vi "sombrero.vi"() -> ()   [LabVIEW 2011]
uses:
  <vilib>/Math Plots/3D Math Plots/3D Surface/3D Surface XCtrl/3D Surface.xctl
  <vilib>/Math Plots/3D Math Plots/3D Surface/3D Surface Datatype/Public/Plot Helper (Vector).vi
  <vilib>/Math Plots/3D Math Plots/3D Surface/3D Surface Datatype/3D Surface Datatype.lvclass
panel:
  in  "Animaatio":bool
  in  "Voimakkuus":dbl(knob) scale=1.1..200.0
  in  "Aallonpituus":dbl(knob) scale=1.1..30.0
  out "3D Surface":refnum<class "3D Plot Datatype.lvclass">[](xcontrol)
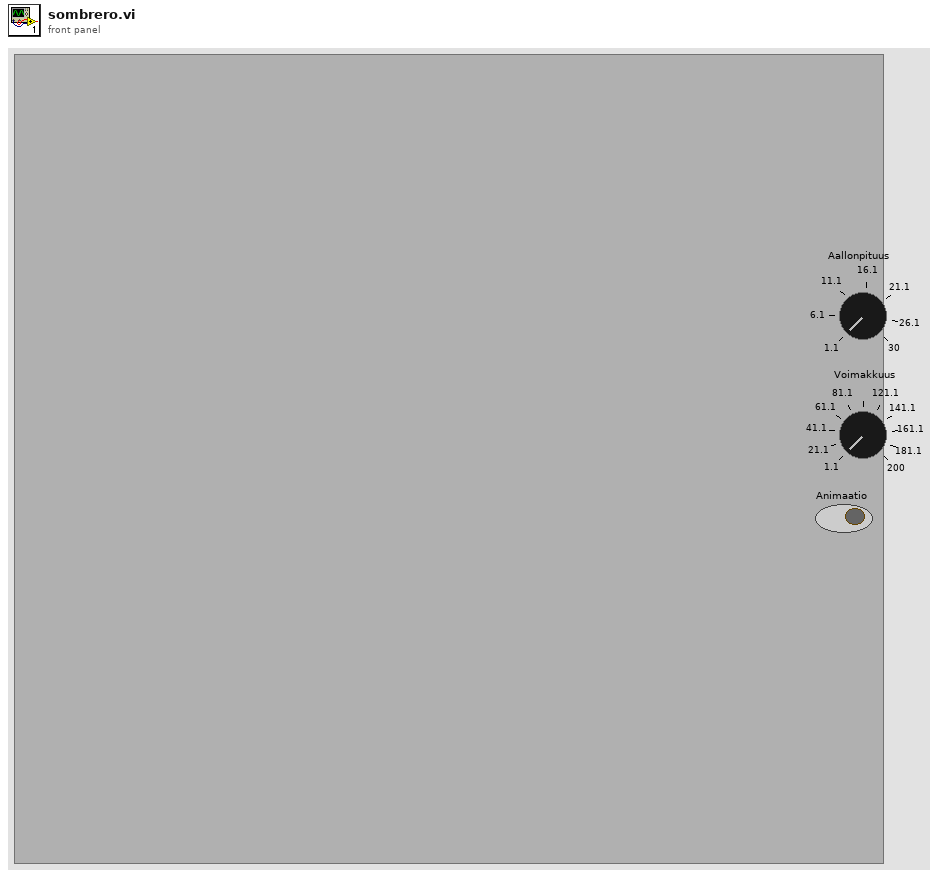
[diagram p1: front panel]
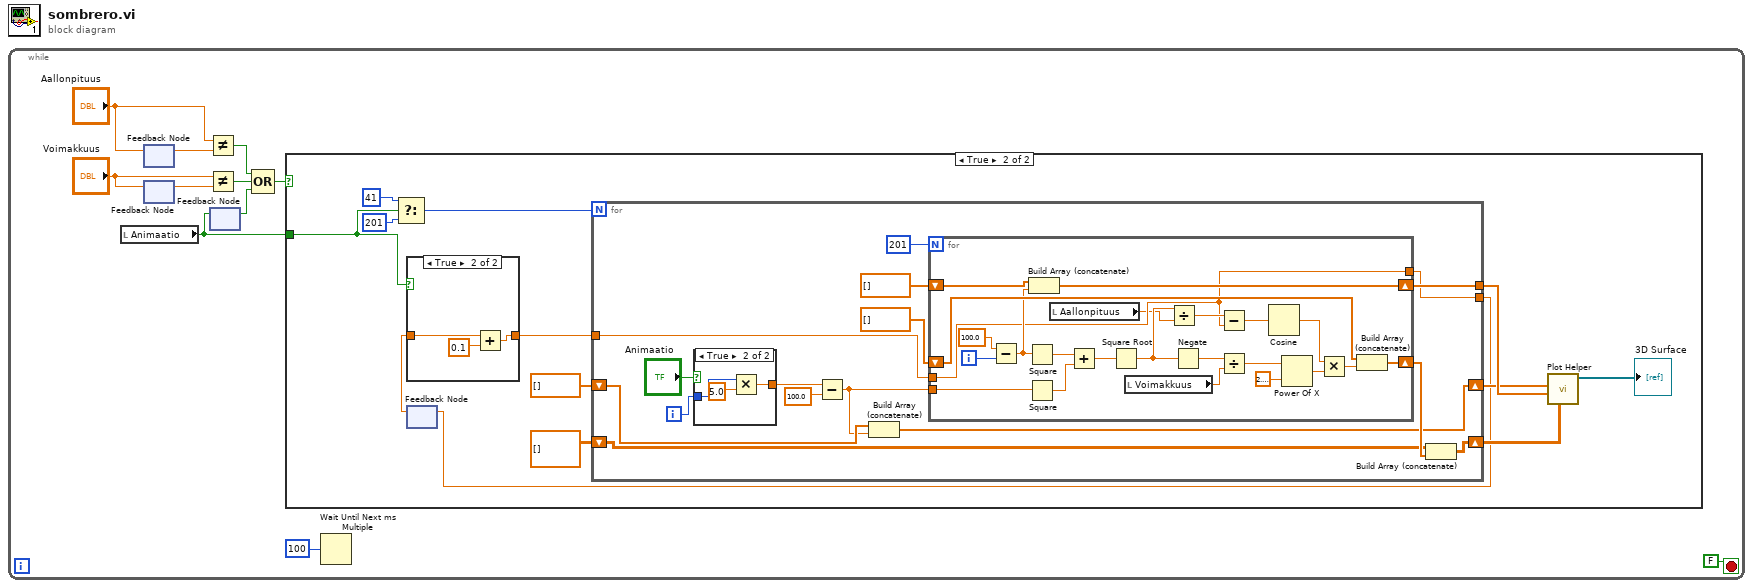
[diagram p0: block diagram]
diagram:
  n1 = while {
    stop <- FALSE stop-if-true
    n2 = local read "Animaatio"() -> (w5:bool)
    n3 = feedback-in #1("Aallonpituus") -> ()
    n4 = feedback #1() -> (w7:dbl)  [unwired: 1 in]
    n5 = feedback-in #2("Voimakkuus") -> ()
    n6 = feedback #2() -> (w9:dbl)  [unwired: 1 in]
    n7 = Not Equal?(x="Aallonpituus", y=w7) -> (x != y?=w4:bool)
    n8 = Not Equal?(x="Voimakkuus", y=w9) -> (x != y?=w3:bool)
    n9 = feedback-in #3(w5) -> ()
    n10 = feedback #3() -> (w2:bool)  [unwired: 1 in]
    n11 = Compound Arithmetic op=OR(w4, w3, w2) -> (w1:bool)
    n12 = case shown="True" w1 {
      tunnel: w5 -> [_ w16]
      frame False {
      }
      frame True {
        n13 = Select(t=41, s=w16, f=201) -> (s? t:f=w17:i32)
        n14 = feedback #4() -> (w12:dbl)  [unwired: 1 in]
        n15 = case shown="True" w16 {
          tunnel: [w25 w27] -> w20
          tunnel: w12 -> [w25 w26]
          frame False {
          }
          frame True {
            n16 = Add(x=w26, y=0.1) -> (x+y=w27:dbl)
          }
        }
        n17 = for {
          N: w17 -> [_]
          tunnel: [w38] -> w22
          shift-right: [w39] -> w23
          shift-left: dbl[][] [] -> [w42]
          tunnel: w20 -> [w37]
          tunnel: [w36] -> w13
          shift-right: [w34] -> w21
          shift-left: dbl[] [] -> [w35]
          i -> [w33]
          n18 = case shown="True" "Animaatio" {
            tunnel: w33 -> [w45 w47]
            tunnel: [w45 w46] -> w31
            frame False {
            }
            frame True {
              n19 = Multiply(x=w47, y=5.0) -> (x*y=w46:dbl)
            }
          }
          n20 = Subtract(x=w31, y=100.0) -> (x-y=w30:dbl)
          n21 = Build Array (concatenate)(w35, w30) -> (w34:dbl[])
          n22 = for {
            N: 201 -> [_]
            tunnel: w30 -> [w55]
            shift-right: [w66] -> w38
            shift-left: dbl[] [] -> [w65]
            shift-right: [w63] -> w43
            shift-left: dbl[] [] -> [w64]
            tunnel: w37 -> [w53]
            tunnel: [w53] -> w36
            i -> [w60]
            n23 = Subtract(x=100.0, y=w60) -> (x-y=w56:dbl)
            n24 = Square(x=w56) -> (x^2=w71:dbl)
            n25 = Square(x=w55) -> (x^2=w59:dbl)
            n26 = Build Array (concatenate)(w65, w56) -> (w66:dbl[])
            n27 = local read "Aallonpituus"() -> (w49:dbl)
            n28 = Add(x=w71, y=w59) -> (x+y=w70:dbl)
            n29 = Square Root(x=w70) -> (sqrt(x)=w68:dbl)
            n30 = local read "Voimakkuus"() -> (w51:dbl)
            n31 = Divide(x=w68, y=w49) -> (x/y=w54:dbl)
            n32 = Negate(x=w68) -> (-x=w69:dbl)
            n33 = Subtract(x=w54, y=w53) -> (x-y=w52:dbl)
            n34 = Divide(x=w69, y=w51) -> (x/y=w62:dbl)
            n35 = Cosine(x=w52) -> (cos(x)=w57:dbl)
            n36 = Power Of X(1:2.718281828459045, 2:w62) -> (0:w67:dbl)
            n37 = Multiply(x=w57, y=w67) -> (x*y=w58:dbl)
            n38 = Build Array (concatenate)(w64, w58) -> (w63:dbl[])
          }
          n39 = Build Array (concatenate)(w42, w43) -> (w39:dbl[][])
        }
        n40 = feedback-in #4(w13) -> ()
        n41 = call-poly <vilib>:"Plot Helper.vi"("z matrix"=w23, "y vector"=w22, "x vector"=w21) -> ("3D Plot lvclass Array out"=→"3D Surface":refnum<class "3D Plot Datatype.lvclass">[])  [unwired: 3 in, 5 out]
      }
    }
    n42 = Wait Until Next ms Multiple(millisecond multiple=u32 100) -> ()  [unwired: 1 out]
  }
